vi "Send Create Channel Arbitrary Waveform I32 [ACH].vi"(7 "Message Priority (Normal)":T1=enum."Normal", 8 "error in (no error)":errorcluster, 9 "Waveform Data Array":i32[](array[numeric]) caption="waveform data array", 10 "Channel Name (\"\")":string="CHANNEL1" caption="channel name (\"CHANNEL1\")", 11 "Message Enqueuer":refnum<class "Message Enqueuer.lvclass">) -> (0 "error out":errorcluster, 3 "Message Enqueuer out":refnum<class "Message Enqueuer.lvclass">)   [LabVIEW 2015, in "CS++Fgen.lvlib" / "Create Channel Arbitrary Waveform I32 [ACH] Msg.lvclass"]
doc: "Sends the <B>CS++Fgen.lvlib:Create Channel Arbitrary Waveform I32 [ACH] Msg.lvclass</B> message.\n\n<B>CS++Fgen.lvlib:CS++Fgen.lvclass:Create Channel Arbitrary Waveform I32 [ACH].vi</B> Description:\n\nThis VI creates a channel-specific arbitrary waveform and returns a handle that identifies that waveform. Data is passed in as 32-bit binary data. If the arbitrary waveform generator supports formats smaller than 32 bits, read the IviFgen Binary Alignment [AB] property to determine whether to left or right justify the data before passing it to this call. \n\nYou pass this handle to the IviFgen Configure Arbitrary Waveform [ARB] VI to produce that waveform. You also use the handles this VI returns to specify a sequence of arbitrary waveforms with the IviFgen Create Arbitrary Sequence [SEQ] VI.\n\nIf the instrument does not support channel-based arbitrary waveform creation, use IviFgen Create Arbitrary Waveform VI.\n\nUse the IviFgen Create Channel Arbitrary Waveform Int16 [AB] VI to create a channel-specific arbitrary waveform if you want to pass data in 16-bit binary. Use the IviFgen Create Channel Arbitrary Waveform [ACH] VI to create a channel-specific arbitrary waveform with normalized data.\n\nNote:\n\n(1) This VI is part of the IviFgenArbWfmBinary [AB] extension group."
uses:
  Create Channel Arbitrary Waveform I32 [ACH] Msg.lvclass
  <vilib>/ActorFramework/Message Enqueuer/Message Enqueuer.lvclass
  <vilib>/ActorFramework/Message Enqueuer/Message Priority.ctl
  Create Channel Arbitrary Waveform I32 [ACH] Msg.lvclass/Create Channel Arbitrary Waveform I32 [ACH] Msg.ctl
  <vilib>/ActorFramework/Message Enqueuer/Message Enqueuer.lvclass/Message Enqueuer.ctl
  <vilib>/ActorFramework/Message Priority Queue/Priority Enqueue.vi
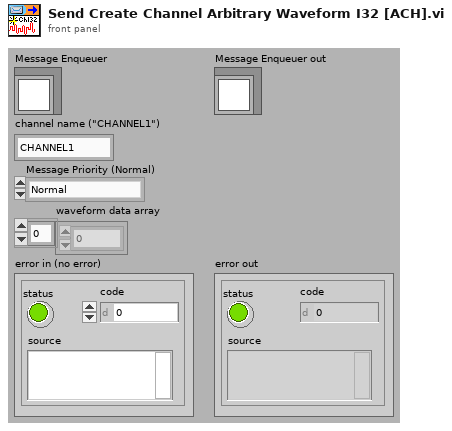
[diagram p1: front panel]
types:
  T1 = typedef "Actor Framework.lvlib/Message Enqueuer.lvclass/Message Priority.ctl" = enum16{"Low", "Normal", "High"}
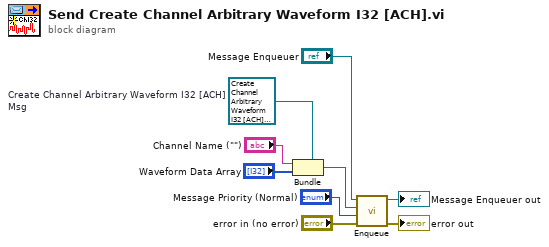
[diagram p0: block diagram]
diagram:
  w3 = refnum<class "Create Channel Arbitrary Waveform I32 [ACH] Msg.lvclass"> refnum  # Create Channel Arbitrary Waveform I32 [ACH] Msg
  n1 = Bundle(cluster=w3, "Channel Name (\"\")", "Waveform Data Array") -> (w6:refnum<class "Create Channel Arbitrary Waveform I32 [ACH] Msg.lvclass">)
  n2 = call <vilib>:"Enqueue.vi"("error in (no error)"="error in (no error)", "Message Priority (Normal)"="Message Priority (Normal)", "Message"=w6, "Message Enqueuer in"="Message Enqueuer") -> ("error out"=→"error out":errorcluster, "Message Enqueuer out"=→"Message Enqueuer out":refnum<class "Message Enqueuer.lvclass">)  [unwired: 6 in]
